vi "LSX Get Power Amplifier.vi"(8 "error in (no error)":errorcluster, 10 "pbAmplifier":i32, 11 "lLSID":i32) -> (0 "error out":errorcluster, 2 "pbAmplifier out":i32, 3 "function return":i32)   [LabVIEW 2018, in "Tango.lvlib"]
doc: "TANGOAPI int TANGOCALL LSX_GetPowerAmplifier (int lLSID, BOOL *pbAmplifier);"
uses:
  Tango.lvlib
  SubVIs/Tango_DLL.dll
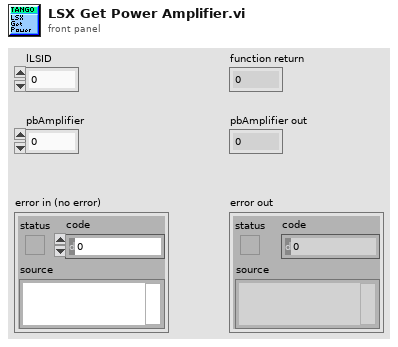
[diagram p1: front panel]
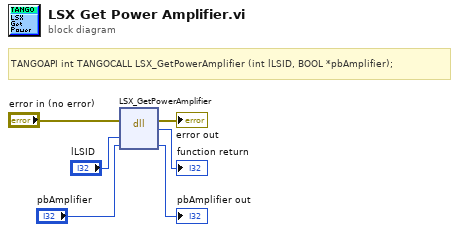
[diagram p0: block diagram]
diagram:
  # "TANGOAPI int TANGOCALL LSX_GetPowerAmplifier (int lLSID, BOOL *pbAmplifier);"
  n1 = dll-call lib="C:/Users/Familie/Documents/LabviewIX81/lib/TANGO Stage/SubVIs/Tango_DLL.*" fn="LSX_GetPowerAmplifier"(error in="error in (no error)", "lLSID"="lLSID", "pbAmplifier"="pbAmplifier") -> (error out=→"error out":errorcluster, →"function return":i32, "pbAmplifier"=→"pbAmplifier out":i32)  [unwired: 3 in, 1 out]
